vi "Add Point.vi"(8 "error in (no error)":errorcluster caption="错误输入（无错误）", 9 "point":cluster{"x":i16, "y":i16} caption="点", 10 "Key":string, 11 "Dictionary In":refnum<class "Dictionary.lvclass"> caption="DNL_LabVIEW Object in") -> (0 "error out":errorcluster caption="错误输出", 1 "Key Exist?":bool, 3 "Dictionary Out":refnum<class "Dictionary.lvclass"> caption="DNL_LabVIEW Object out")   [LabVIEW 2012, in "Dictionary.lvclass"]
uses:
  Dictionary.lvclass
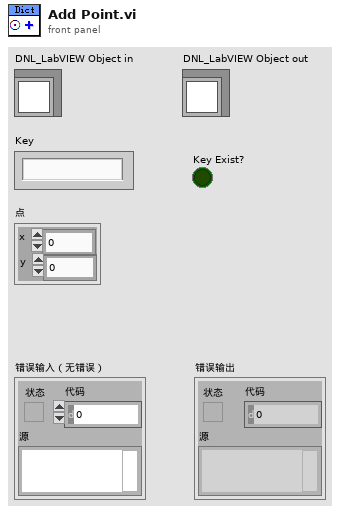
[diagram p1: front panel]
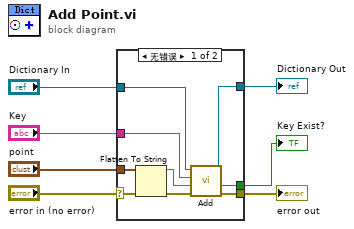
[diagram p0: block diagram]
diagram:
  n1 = case shown="无错误" "error in (no error)" {
    selector: "error in (no error)" -> [w15 w18]
    tunnel: [w8 w18] -> w6
    tunnel: [w12 w17] -> w4
    tunnel: "Dictionary In" -> [w13 w17]
    tunnel: "point" -> [w16 _]
    tunnel: [w11 _] -> w2
    tunnel: "Key" -> [w9 _]
    frame No Error {
      n2 = Flatten To String(anything=w16, error in (no error)=w15) -> (data string=w10:string, error out=w14:errorcluster)  [unwired: 2 in, 1 out]
      n3 = call "Add.vi"("error in (no error)"=w14, "Value"=w10, "Key"=w9, "Dictionary In"=w13) -> ("error out"=w8:errorcluster, "Key Exist?"=w11:bool, "Dictionary Out"=w12:refnum<class "Dictionary.lvclass">)  [unwired: 5 in]
    }
    frame Error {
    }
  }
  "error out" <- w6
  "Dictionary Out" <- w4
  "Key Exist?" <- w2
